vi "Read UID.vi"(8 "error in":errorcluster, 11 "configuration in":refnum<class "NISE_CEF_serializable configuration.lvclass">) -> (0 "error out":errorcluster, 2 "instance id":string, 3 "configuration out":refnum<class "NISE_CEF_serializable configuration.lvclass">)   [LabVIEW 2013, in "NISE_CEF_serializable configuration.lvclass"]
doc: "Provides the instance name of a given configuration/runtime class pairing. This instance may be used as an identifier to differentiate between configurations. On first call, this instance ID is generated."
uses:
  NISE_CEF_serializable configuration.lvclass
  NISE_CEF_serializable configuration.lvclass/NISE_CEF_serializable configuration.ctl
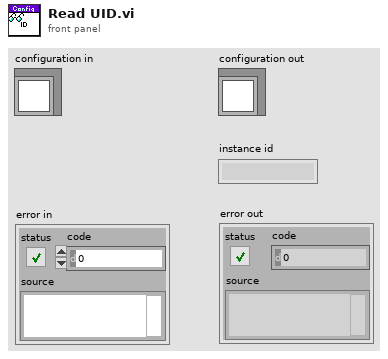
[diagram p1: front panel]
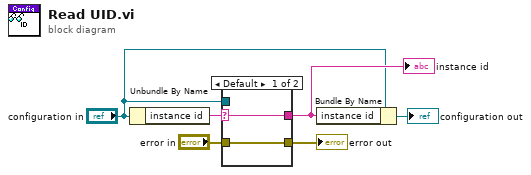
[diagram p0: block diagram]
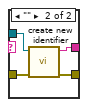
[diagram p2: hidden frame]
diagram:
  n1 = Unbundle By Name("configuration in") -> ("instance id"=w4:string)
  n2 = case shown="Default" w4 {
    selector: w4 -> [w8 _]
    tunnel: [w8 w11] -> w5
    tunnel: "configuration in" -> [_ w12]
    tunnel: [w7 w10] -> w2
    tunnel: "error in" -> [w7 w9]
    frame Default {
    }
    frame "" {
      n3 = call-dynamic "create new identifier.vi"("error in"=w9, "configuration in"=w12) -> ("error out"=w10:errorcluster, "id"=w11:string)  [unwired: 8 in]
    }
  }
  "instance id" <- w5
  "error out" <- w2
  n4 = Bundle By Name(cluster="configuration in", "instance id"=w5) -> (→"configuration out":refnum<class "NISE_CEF_serializable configuration.lvclass">)
